vi "Update MotorV SP in MeasDataQ.vi"(8 "error in (no error)":errorcluster, 9 "TimeStamp":timestamp, 10 "MotorV SP":dbl) -> (0 "error out":errorcluster, 3 "orData out":T1)   [LabVIEW 2017]
doc: "Developed by Kevin Thompson\nThompson Engineering, LLC\nkevin@thompsonengineering.net"
uses:
  TD MeasData QRef.ctl
  TD MeasData--cluster.ctl
  GBL DataQ Ref.vi
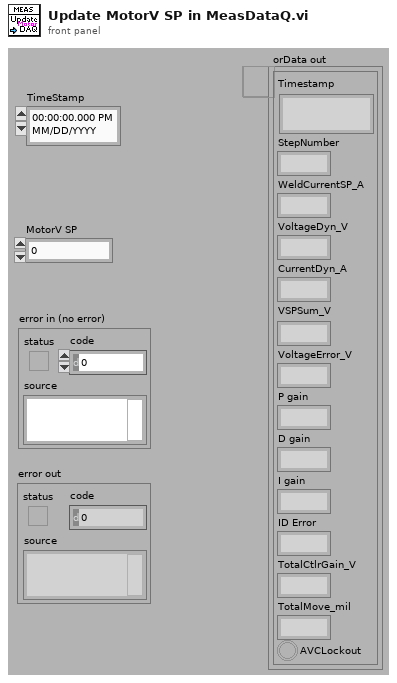
[diagram p1: front panel]
types:
  T1 = typedef "TD MeasData QRef.ctl" = refnum<queue>
  T2 = typedef "TD MeasData--cluster.ctl" = cluster{"Timestamp":timestamp, "StepNumber":i32, "WeldCurrentSP_A":dbl, "VoltageDyn_V":dbl, "CurrentDyn_A":dbl, "VSPSum_V":dbl, "VoltageError_V":dbl, "P gain":dbl, "D gain":dbl, "I gain":dbl, "ID Error":dbl, "TotalCtlrGain_V":dbl, "TotalMove_mil":dbl, "AVCLockout":bool}
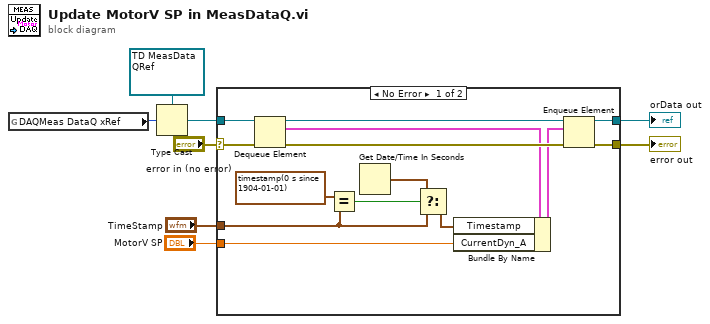
[diagram p0: block diagram]
diagram:
  n1 = global read "GBL DataQ Ref.vi" "DAQMeas DataQ xRef"() -> (w2:u32)
  n2 = Type Cast(type=T1 refnum ("orData in"), x=w2) -> (*(type *) &x=w4:T1)
  n3 = case shown="No Error" "error in (no error)" {
    selector: "error in (no error)" -> [w17 w23]
    tunnel: w4 -> [w22 w24]
    tunnel: [w19 w23] -> w8
    tunnel: [w18 w24] -> w7
    tunnel: "TimeStamp" -> [w11 _]
    tunnel: "MotorV SP" -> [w14 _]
    frame No Error {
      n4 = Dequeue Element(queue=w22, error in (no error)=w17) -> (queue out=w20:T1, element=w16:T2, error out=w21:errorcluster)  [unwired: 1 in, 1 out]
      n5 = Equal?(x=timestamp(0 s since 1904-01-01) ("TimeStamp"), y=w11) -> (x = y?=w12:bool)
      n6 = Get Date/Time In Seconds() -> (seconds since 1Jan1904=w9:timestamp)
      n7 = Select(t=w9, s=w12, f=w11) -> (s? t:f=w10:timestamp)
      n8 = Bundle By Name(cluster=w16, "Timestamp"=w10, "CurrentDyn_A"=w14) -> (w15:T2)
      n9 = Enqueue Element(queue=w20, element=w15, error in (no error)=w21) -> (queue out=w18:T1, error out=w19:errorcluster)  [unwired: 1 in, 1 out]
    }
    frame Error {
    }
  }
  "orData out" <- w7
  "error out" <- w8
